vi "OilValveTiming.vi"(0 "FPGA VI Reference In":refnum<k20>, 1 "reference":refnum<vi>, 3 "host loop update rate":u32, 5 "error in":errorcluster, 7 "stop in":bool) -> (6 "Waveform Graph":dbl[](graph), 10 "x > y?":bool, 11 "x .and. y?":bool, 12 "Elements Remaining 2":u32, 13 "FPGA VI Reference Out":refnum<k20>, 14 "Waveform Graph 2":waveform(dbl)[](graph), 15 "Data FIFO Full 2":bool, 16 "x .and. y? 2":bool, 17 "x > y? 2":bool, 18 "Host error out 2":errorcluster, 19 "error out":errorcluster)   [LabVIEW 2017]
uses:
  <vilib>/Utility/error.llb/Error Cluster From Error Code.vi
  <vilib>/rvi/errors/niLvFpgaAdjustHostInterfaceError.vi
  <vilib>/measure/madcrms.llb/Basic Averaged DC-RMS for N Chan.vi
  <vilib>/rvi/interface/nirviMethod/nirviMethod.xnode
  FPGA Bitfiles/80Ton_FPGATarget_accelerometer_vQr4SS40msc.lvbitx
  FPGA Bitfiles/accelerometer.vi
  <vilib>/rvi/interface/nirviReadWriteControl/nirviReadWriteControl.xnode
  <vilib>/measure/NI_MAPro.lvlib
  <vilib>/FPGAPlugInAG/cRIO-9035/niLvFpga_ReadFifo_cRIO-9035.vi
  <vilib>/rvi/errors/niLvFpgaMergeErrorWithErrorCode.vi
  NiFpgaLv.dll
panel:
  out "Waveform Graph 4":dbl[](graph)
  out "RMS values 2":dbl[](array[numeric]) format="%.2p"
  out "Waveform Graph 3":waveform(dbl)[](graph)
  in  "stop in 2":bool
  out "Numeric 2":i32
  out "Numeric":i32
  in  "Open":bool
  out "RMS values":dbl[](array[numeric]) format="%.2p"
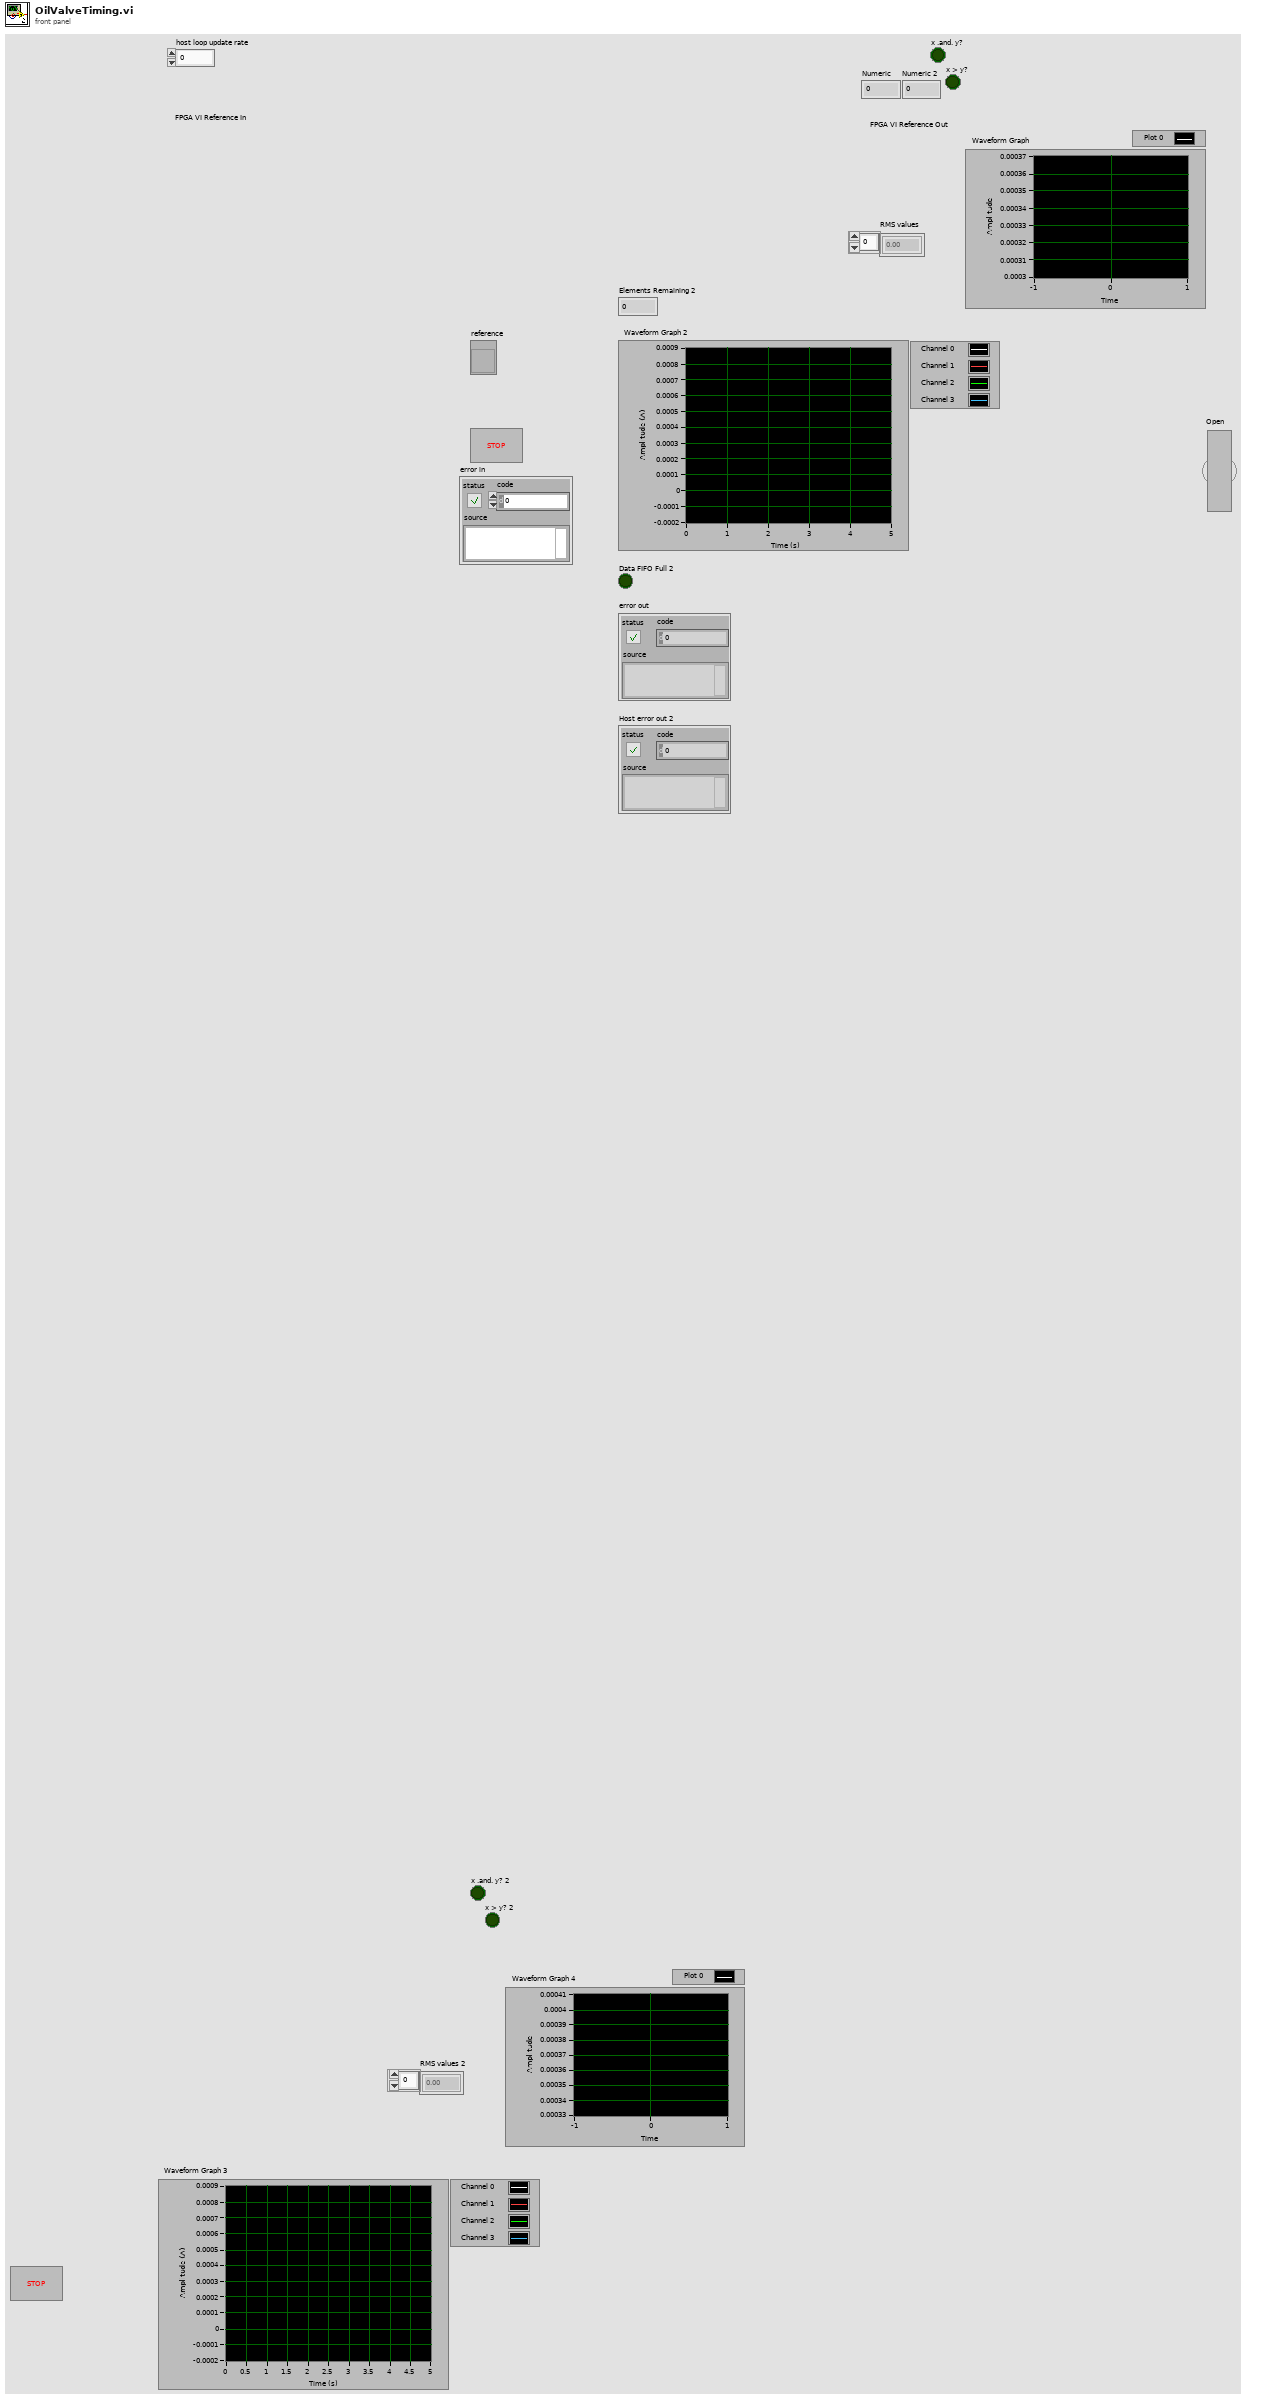
[diagram p1: front panel]
types:
  T1 = enum16{"Rectangular (none)", "Hanning", "Low side lobe"}
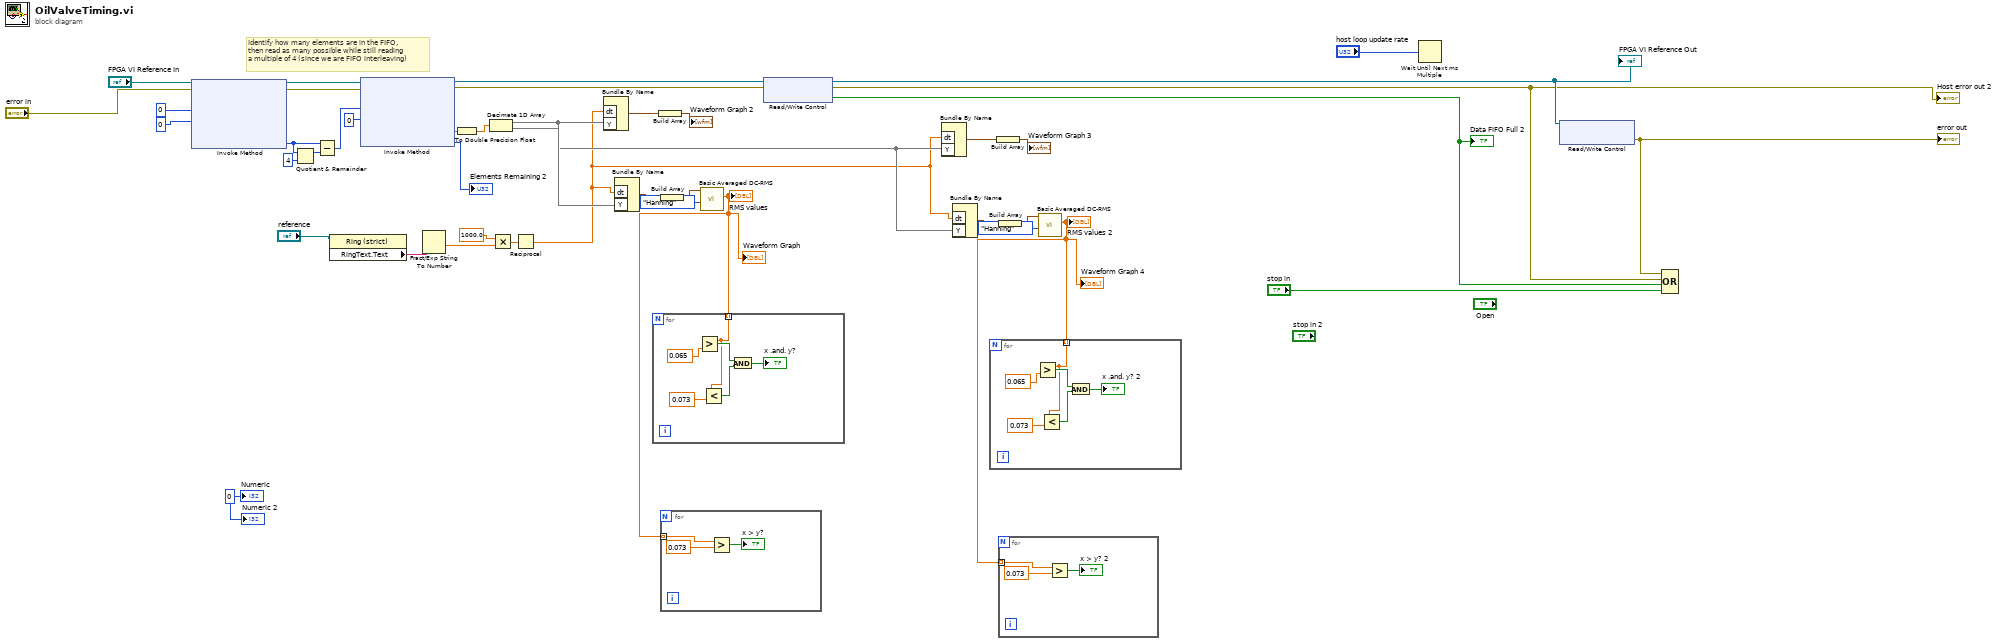
[diagram p0: block diagram]
diagram:
  w10 = 0
  # "Identify how many elements are in the FIFO, \nthen read as many possible while still reading\na multiple of 4 (since we are FIFO interleaving)"
  n1 = xnode "Invoke Method"("FPGA VI Reference In"="FPGA VI Reference In", "error in"="error in", "Number of Elements"=u32 0, "Timeout (ms)"=0) -> ("FPGA VI Reference Out"=w40:refnum<k20>, "error out"=w39:errorcluster, "Elements Remaining"=w14:u32)  [unwired: 1 out]
  n2 = Quotient & Remainder(x=w14, y=u32 4) -> (x-y*floor(x/y)=w42:u32)  [unwired: 1 out]
  n3 = Subtract(x=w14, y=w42) -> (x-y=w43:u32)
  n4 = property on="Property Node" class="Ring (strict)"(reference="reference") -> ("RingText.Text"=w34:string)  [unwired: 1 in, 2 out]
  n5 = xnode "Invoke Method"("FPGA VI Reference In"=w40, "error in"=w39, "Number of Elements"=w43, "Timeout (ms)"=0 ("Timeout")) -> ("FPGA VI Reference Out"=w31:refnum<k20>, "error out"=w32:errorcluster, "Data"=w30:fxp<+/-,24,5>[], "Elements Remaining"=→"Elements Remaining 2":u32)
  n6 = Fract/Exp String To Number(string=w34) -> (number=w27:dbl)  [unwired: 4 out]
  n7 = To Double Precision Float(number=w30) -> (double precision float=w36:dbl[])
  n8 = Decimate 1D Array(w36) -> (w20:dbl[], w2:dbl[])
  n9 = Multiply(x=1000.0, y=w27) -> (x*y=w28:dbl)
  n10 = Reciprocal(x=w28) -> (1/x=w1:dbl)
  n11 = Bundle By Name("dt"=w1, "Y"=w20) -> (w35:waveform(dbl))  [unwired: 1 out]
  n12 = Bundle By Name("dt"=w1, "Y"=w20) -> (w19:waveform(dbl))  [unwired: 1 out]
  n13 = Build Array(w35) -> (→"Waveform Graph 2":waveform(dbl)[])
  n14 = Build Array(w19) -> (w18:waveform(dbl)[])
  n15 = call-poly <vilib>:"Basic Averaged DC-RMS.vi"("window"=T1."Hanning", "signals in"=w18) -> ("RMS values"=w11:dbl[])  [unwired: 6 in, 3 out]
  "RMS values" <- w11
  "Waveform Graph" <- w11
  n16 = for {
    tunnel: w11 -> [w47] mode=indexing
    n17 = Greater?(x=w47, y=0.065) -> (0:w48:bool)
    n18 = Less?(x=w47, y=0.073) -> (x < y?=w45:bool)
    n19 = And(x=w48, y=w45) -> (x .and. y?=→"x .and. y?":bool)
  }
  n20 = for {
    tunnel: w11 -> [w51] mode=indexing
    n21 = Greater?(x=w51, y=0.073) -> (0:→"x > y?":bool)
  }
  n22 = xnode "Read/Write Control"("FPGA VI Reference In"=w31, "error in"=w32) -> ("FPGA VI Reference Out"=w23:refnum<k20>, "error out"=w13:errorcluster, "Data FIFO Full"=w38:bool)
  "Host error out 2" <- w13
  "Data FIFO Full 2" <- w38
  "FPGA VI Reference Out" <- w23
  n23 = Bundle By Name("dt"=w1, "Y"=w2) -> (w8:waveform(dbl))  [unwired: 1 out]
  n24 = Bundle By Name("dt"=w1, "Y"=w2) -> (w6:waveform(dbl))  [unwired: 1 out]
  n25 = Build Array(w8) -> (→"Waveform Graph 3":waveform(dbl)[])
  n26 = Build Array(w6) -> (w5:waveform(dbl)[])
  n27 = call-poly <vilib>:"Basic Averaged DC-RMS.vi"("window"=T1."Hanning", "signals in"=w5) -> ("RMS values"=w3:dbl[])  [unwired: 6 in, 3 out]
  "RMS values 2" <- w3
  "Waveform Graph 4" <- w3
  n28 = for {
    tunnel: w3 -> [w56] mode=indexing
    n29 = Greater?(x=w56, y=0.065) -> (0:w57:bool)
    n30 = Less?(x=w56, y=0.073) -> (x < y?=w54:bool)
    n31 = And(x=w57, y=w54) -> (x .and. y?=→"x .and. y? 2":bool)
  }
  n32 = for {
    tunnel: w3 -> [w60] mode=indexing
    n33 = Greater?(x=w60, y=0.073) -> (0:→"x > y? 2":bool)
  }
  n34 = Wait Until Next ms Multiple(millisecond multiple="host loop update rate") -> ()  [unwired: 1 out]
  n35 = xnode "Read/Write Control"("FPGA VI Reference In"=w23) -> ("FPGA Error Out"=w24:errorcluster)  [unwired: 1 in, 2 out]
  "error out" <- w24
  n36 = Compound Arithmetic op=OR(w24, w13, w38, "stop in") -> ()  [unwired: 1 out]
  "Numeric" <- w10
  "Numeric 2" <- w10
